vi "Statistics Calculations.vi"(6 "error in":errorcluster, 7 "GlobalData":T1, 11 "Time Array":i32[][](array[numeric])) -> (3 "Time Array":i32[][](array[numeric]), 4 "error out":errorcluster)   [LabVIEW 2024]
doc: "Data Statistics"
uses:
  controls/GlobalData.ctl
  <vilib>/Analysis/baseanly.llb/Unimode.vi
  <vilib>/Analysis/NI_AALBase.lvlib
  <vilib>/gmath/NI_Gmath.lvlib
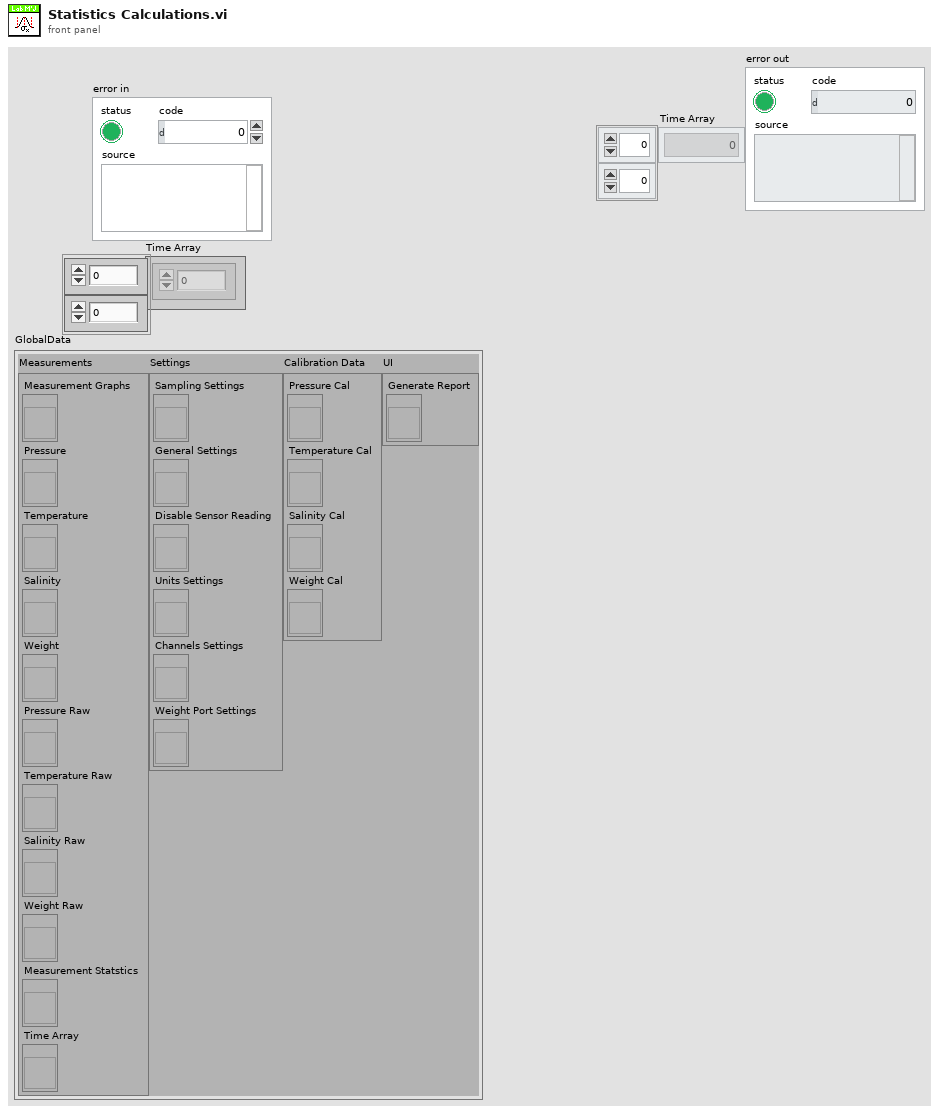
[diagram p1: front panel]
types:
  T1 = typedef "GlobalData.ctl" = cluster{"Measurements":cluster{"Measurement Graphs":refnum<vi>, "Pressure":refnum<vi>, "Temperature":refnum<vi>, "Salinity":refnum<vi>, "Weight":refnum<vi>, "Pressure Raw":refnum<vi>, "Temperature Raw":refnum<vi>, "Salinity Raw":refnum<vi>, "Weight Raw":refnum<vi>, "Measurement Statstics":refnum<vi>, "Time Array":refnum<vi>}, "Settings":cluster{"Sampling Settings":refnum<vi>, "General Settings":refnum<vi>, "Disable Sensor Reading":refnum<vi>, "Units Settings":refnum<vi>, "Channels Settings":refnum<vi>, "Weight Port Settings":refnum<vi>}, "Calibration Data":cluster{"Pressure Cal":refnum<vi>, "Temperature Cal":refnum<vi>, "Salinity Cal":refnum<vi>, "Weight Cal":refnum<vi>}, "UI":cluster{"Generate Report":refnum<vi>}}
  T2 = cluster{"Reading Time (ms)":u64, "Graph Time ":u16}
  T3 = cluster{"Pressure":dbl[], "Temperature":dbl[], "Salinity":dbl[], "Weight":dbl[]}
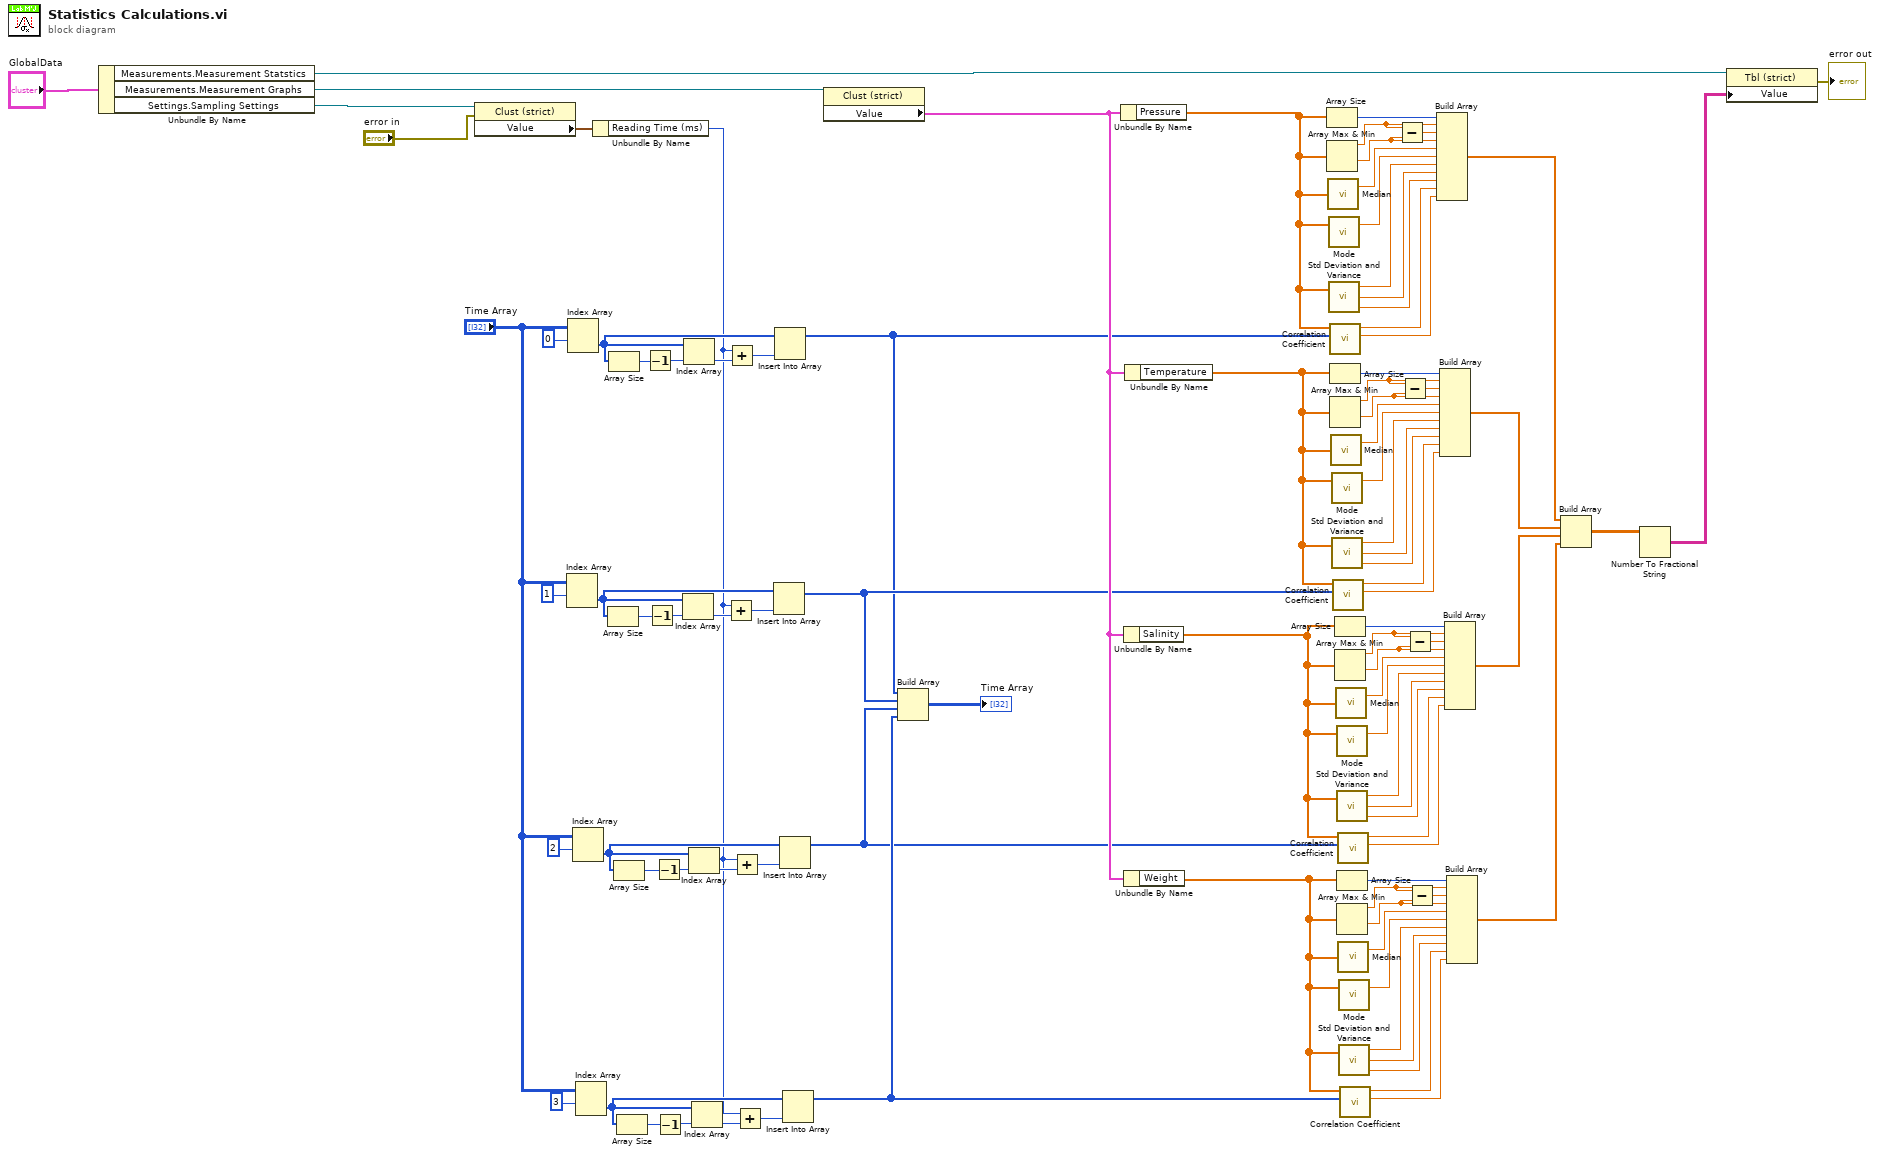
[diagram p0: block diagram]
diagram:
  n1 = Unbundle By Name("GlobalData") -> ("Measurements.Measurement Statstics"=w93:refnum<vi>, "Measurements.Measurement Graphs"=w92:refnum<vi>, "Settings.Sampling Settings"=w85:refnum<vi>)
  n2 = property class="Clust (strict)"(reference=w85, error in="error in") -> ("Value"=w84:T2)  [unwired: 2 out]
  n3 = Index Array(array="Time Array", index (row)=1 ("disabled index (col)")) -> (element=w35:i32[])  [unwired: 1 in]
  n4 = Index Array(array="Time Array", index (row)=0 ("disabled index (col)")) -> (element=w38:i32[])  [unwired: 1 in]
  n5 = Index Array(array="Time Array", index (row)=2 ("disabled index (col)")) -> (element=w30:i32[])  [unwired: 1 in]
  n6 = Index Array(array="Time Array", index (row)=3 ("disabled index (col)")) -> (element=w27:i32[])  [unwired: 1 in]
  n7 = Unbundle By Name(w84) -> ("Reading Time (ms)"=w23:u64)
  n8 = Array Size(array=w35) -> (size(s)=w6:i32)
  n9 = Array Size(array=w38) -> (size(s)=w8:i32)
  n10 = Array Size(array=w30) -> (size(s)=w4:i32)
  n11 = Array Size(array=w27) -> (size(s)=w2:i32)
  n12 = Decrement(x=w8) -> (x-1=w7:i32)
  n13 = Decrement(x=w6) -> (x-1=w5:i32)
  n14 = Decrement(x=w4) -> (x-1=w3:i32)
  n15 = Decrement(x=w2) -> (x-1=w1:i32)
  n16 = Index Array(array=w35, index=w5) -> (element=w34:i32)
  n17 = Index Array(array=w38, index=w7) -> (element=w39:i32)
  n18 = Index Array(array=w30, index=w3) -> (element=w31:i32)
  n19 = Index Array(array=w27, index=w1) -> (element=w26:i32)
  n20 = Add(x=w23, y=w34) -> (x+y=w36:u64)
  n21 = Add(x=w23, y=w39) -> (x+y=w37:u64)
  n22 = Add(x=w23, y=w31) -> (x+y=w29:u64)
  n23 = Add(x=w23, y=w26) -> (x+y=w28:u64)
  n24 = Insert Into Array(array=w35, new element=w36) -> (w20:i32[])  [unwired: 1 in]
  n25 = Insert Into Array(array=w38, new element=w37) -> (w19:i32[])  [unwired: 1 in]
  n26 = Insert Into Array(array=w30, new element=w29) -> (w21:i32[])  [unwired: 1 in]
  n27 = Insert Into Array(array=w27, new element=w28) -> (w22:i32[])  [unwired: 1 in]
  n28 = property class="Clust (strict)"(reference=w92) -> ("Value"=w44:T3)  [unwired: 1 in, 2 out]
  n29 = Build Array(w19, w20, w21, w22) -> (→"Time Array":i32[][])
  n30 = Unbundle By Name(w44) -> ("Pressure"=w86:dbl[])
  n31 = Unbundle By Name(w44) -> ("Salinity"=w43:dbl[])
  n32 = Unbundle By Name(w44) -> ("Weight"=w42:dbl[])
  n33 = Unbundle By Name(w44) -> ("Temperature"=w45:dbl[])
  n34 = Array Size(array=w86) -> (size(s)=w41:i32)
  n35 = Array Max & Min(array=w86) -> (max value=w80:dbl, min value=w79:dbl)  [unwired: 2 out]
  n36 = call <vilib>:"Median.vi"("X"=w86) -> ("median"=w91:dbl)  [unwired: 1 out]
  n37 = call-poly <vilib>:"Mode.vi"("X"=w86) -> ("mode"=w90:dbl)  [unwired: 1 in, 1 out]
  n38 = call <vilib>:"Std Deviation and Variance.vi"("X"=w86) -> ("mean"=w89:dbl, "standard deviation"=w88:dbl, "variance"=w87:dbl)  [unwired: 1 in]
  n39 = call <vilib>:"Correlation Coefficient.vi"("Y"=w19, "X"=w86) -> ("r^2"=w82:dbl, "correlation coefficient r"=w83:dbl)  [unwired: 8 in]
  n40 = Array Size(array=w45) -> (size(s)=w73:i32)
  n41 = Array Max & Min(array=w45) -> (max value=w77:dbl, min value=w78:dbl)  [unwired: 2 out]
  n42 = call <vilib>:"Median.vi"("X"=w45) -> ("median"=w68:dbl)  [unwired: 1 out]
  n43 = call-poly <vilib>:"Mode.vi"("X"=w45) -> ("mode"=w69:dbl)  [unwired: 1 in, 1 out]
  n44 = call <vilib>:"Std Deviation and Variance.vi"("X"=w45) -> ("mean"=w70:dbl, "standard deviation"=w71:dbl, "variance"=w72:dbl)  [unwired: 1 in]
  n45 = call <vilib>:"Correlation Coefficient.vi"("Y"=w20, "X"=w45) -> ("r^2"=w75:dbl, "correlation coefficient r"=w74:dbl)  [unwired: 8 in]
  n46 = Array Size(array=w43) -> (size(s)=w62:i32)
  n47 = Array Max & Min(array=w43) -> (max value=w58:dbl, min value=w57:dbl)  [unwired: 2 out]
  n48 = call <vilib>:"Median.vi"("X"=w43) -> ("median"=w67:dbl)  [unwired: 1 out]
  n49 = call-poly <vilib>:"Mode.vi"("X"=w43) -> ("mode"=w66:dbl)  [unwired: 1 in, 1 out]
  n50 = call <vilib>:"Std Deviation and Variance.vi"("X"=w43) -> ("mean"=w65:dbl, "standard deviation"=w64:dbl, "variance"=w63:dbl)  [unwired: 1 in]
  n51 = Array Size(array=w42) -> (size(s)=w51:i32)
  n52 = Array Max & Min(array=w42) -> (max value=w55:dbl, min value=w56:dbl)  [unwired: 2 out]
  n53 = call <vilib>:"Correlation Coefficient.vi"("Y"=w21, "X"=w43) -> ("r^2"=w60:dbl, "correlation coefficient r"=w61:dbl)  [unwired: 8 in]
  n54 = call <vilib>:"Median.vi"("X"=w42) -> ("median"=w46:dbl)  [unwired: 1 out]
  n55 = call-poly <vilib>:"Mode.vi"("X"=w42) -> ("mode"=w47:dbl)  [unwired: 1 in, 1 out]
  n56 = call <vilib>:"Std Deviation and Variance.vi"("X"=w42) -> ("mean"=w48:dbl, "standard deviation"=w49:dbl, "variance"=w50:dbl)  [unwired: 1 in]
  n57 = call <vilib>:"Correlation Coefficient.vi"("Y"=w22, "X"=w42) -> ("r^2"=w53:dbl, "correlation coefficient r"=w52:dbl)  [unwired: 8 in]
  n58 = Subtract(x=w80, y=w79) -> (x-y=w81:dbl)
  n59 = Subtract(x=w77, y=w78) -> (x-y=w76:dbl)
  n60 = Subtract(x=w58, y=w57) -> (x-y=w59:dbl)
  n61 = Subtract(x=w55, y=w56) -> (x-y=w54:dbl)
  n62 = Build Array(w41, w80, w81, w79, w91, w90, w89, w88, w87, w83, w82) -> (w18:dbl[])
  n63 = Build Array(w73, w77, w76, w78, w68, w69, w70, w71, w72, w74, w75) -> (w15:dbl[])
  n64 = Build Array(w62, w58, w59, w57, w67, w66, w65, w64, w63, w61, w60) -> (w16:dbl[])
  n65 = Build Array(w51, w55, w54, w56, w46, w47, w48, w49, w50, w52, w53) -> (w17:dbl[])
  n66 = Build Array(w18, w15, w16, w17) -> (w13:dbl[][])
  n67 = Number To Fractional String(number=w13) -> (F-format string=w12:string[][])  [unwired: 3 in]
  n68 = property class="Tbl (strict)"(reference=w93, "Value"=w12) -> (error out=→"error out":errorcluster)  [unwired: 1 in, 1 out]
